vi "Write Handle Cluster.vi"(8 "error in (no error)":errorcluster, 10 "Handle Cluster":T1, 11 "Initialize_card in":refnum<class "Control_card.lvclass">) -> (0 "error out":errorcluster, 3 "Initialize_card out":refnum<class "Control_card.lvclass">)   [LabVIEW 2015, in "Control_card.lvclass"]
uses:
  Control_card.lvclass
  Control_card.lvclass/Control_card.ctl
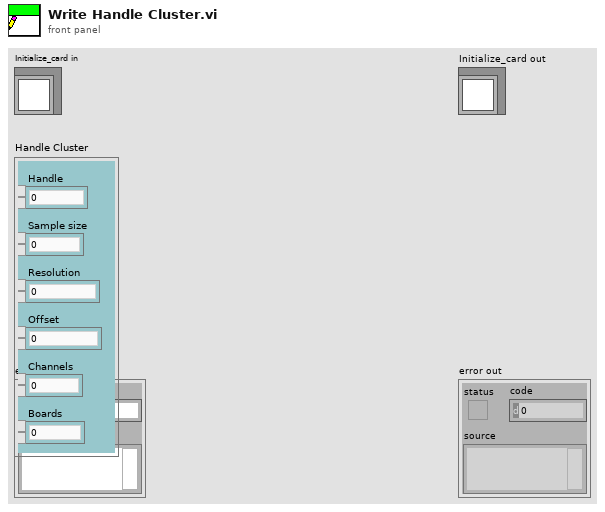
[diagram p1: front panel]
types:
  T1 = cluster{"Handle":u32, "Sample size":u32, "Resolution":i32, "Offset":i32, "Channels":u32, "Boards":u32}
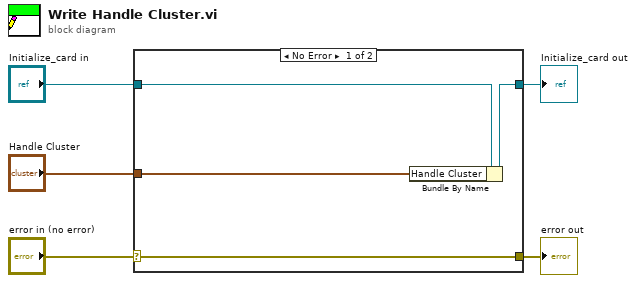
[diagram p0: block diagram]
diagram:
  n1 = case shown="No Error" "error in (no error)" {
    selector: "error in (no error)" -> [w9 w10]
    tunnel: [w9 w10] -> w4
    tunnel: [w7 w11] -> w2
    tunnel: "Initialize_card in" -> [w8 w11]
    tunnel: "Handle Cluster" -> [w6 _]
    frame No Error {
      n2 = Bundle By Name(cluster=w8, "Handle Cluster"=w6) -> (w7:refnum<class "Control_card.lvclass">)
    }
    frame Error {
    }
  }
  "error out" <- w4
  "Initialize_card out" <- w2
